vi "CoinDetector3.vi"() -> ()   [LabVIEW 2020]
uses:
  <vilib>/Analysis/5stat.llb/RMS (DBL).vi
  <vilib>/Analysis/NI_AALPro.lvlib
panel:
  in  "Boolean 3":bool
  in  "Boolean 2":bool
  in  "Boolean":bool
  out "7500 Hz":dbl
  out "6000 Hz":dbl
  out "3000 Hz":dbl
  out "data 2":dynamicdata(graph) caption="data"
  out "data":dynamicdata(graph)
  out "Freq":dbl
  out "Freq 2":dbl
  out "RMS2":dbl
  out "RMS":dbl
  in  "stop":bool
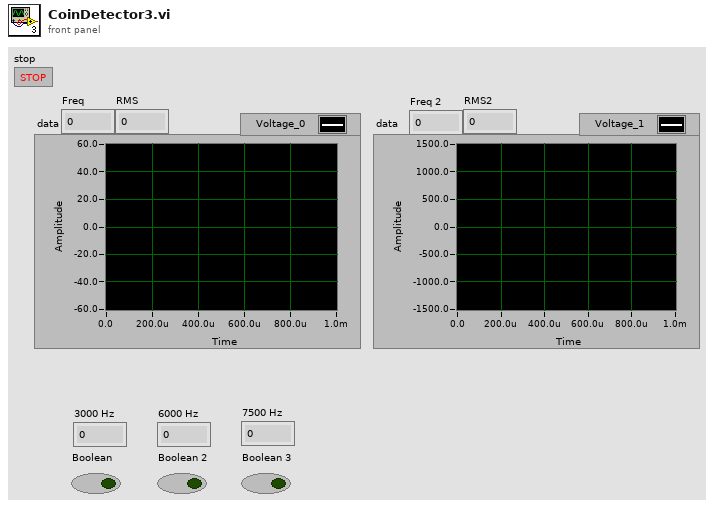
[diagram p1: front panel]
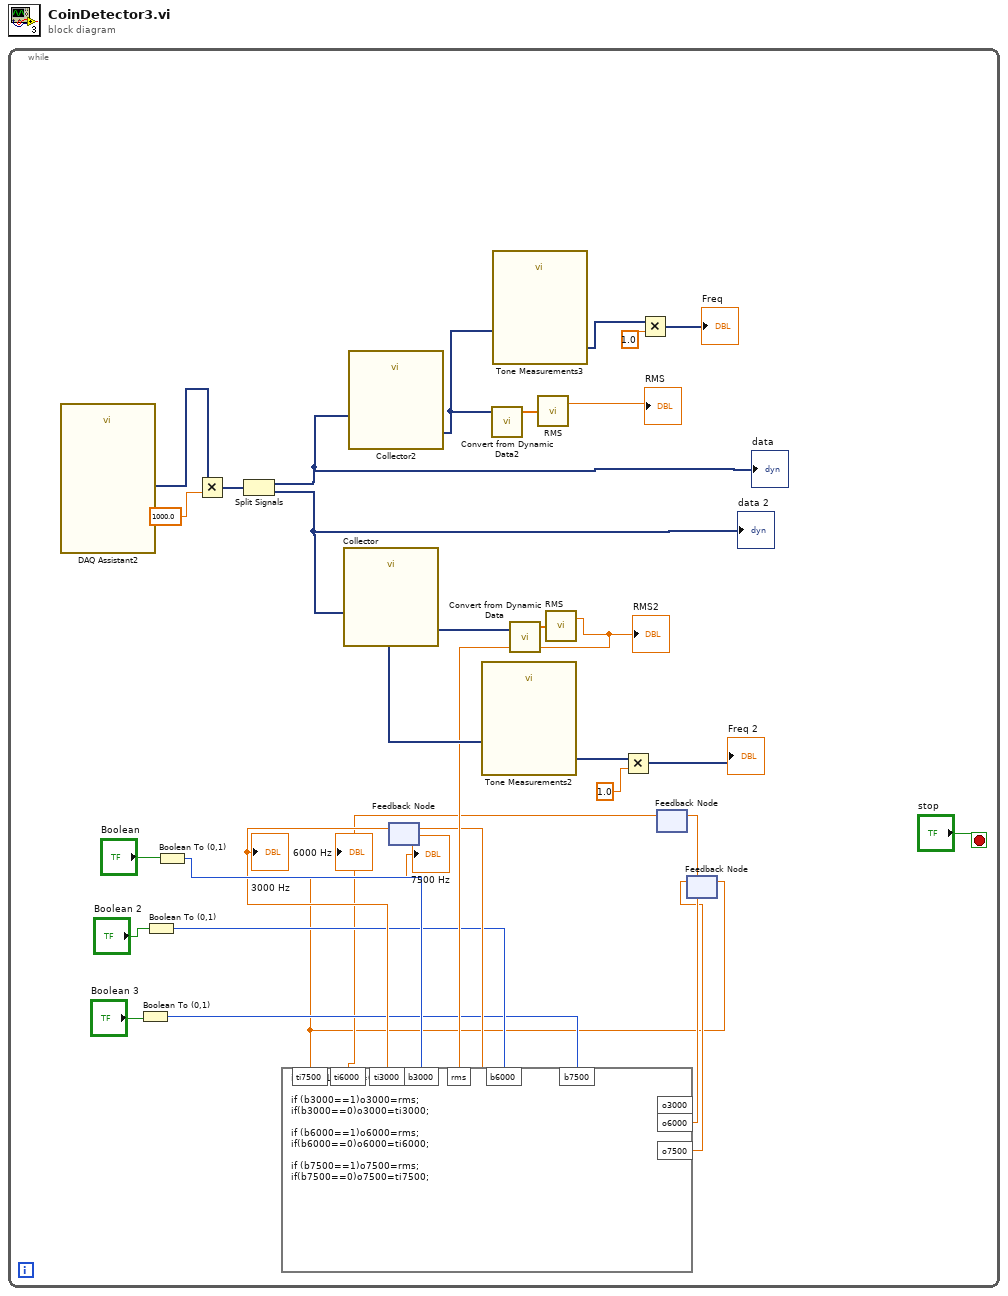
[diagram p0: block diagram]
diagram:
  n1 = while {
    stop <- "stop" stop-if-true
    n2 = call "DAQ Assistant2"() -> ("data"=w18:dynamicdata)  [unwired: 16 in, 3 out]
    n3 = Boolean To (0,1)(Boolean="Boolean 3") -> (0, 1=w5:i16)
    n4 = Boolean To (0,1)(Boolean="Boolean 2") -> (0, 1=w6:i16)
    n5 = Boolean To (0,1)(Boolean="Boolean") -> (0, 1=w12:i16)
    n6 = Multiply(x=w18, y=1000.0) -> (x*y=w28:dynamicdata)
    n7 = Split Signals(w28) -> (w15:dynamicdata, w14:dynamicdata)  [unwired: 2 in]
    "data" <- w15
    "data 2" <- w14
    n8 = call "Collector"("Signals"=w14) -> ("Collected Signals"=w17:dynamicdata)  [unwired: 9 in, 1 out]
    n9 = call "Collector2"("Signals"=w15) -> ("Collected Signals"=w22:dynamicdata)  [unwired: 9 in, 1 out]
    n10 = feedback #1() -> (w9:dbl)  [unwired: 1 in]
    "3000 Hz" <- w9
    n11 = call "Tone Measurements2"("Signals"=w17) -> ("Frequency"=w25:dynamicdata)  [unwired: 9 in, 1 out]
    n12 = call "Convert from Dynamic Data2"("Dynamic Data Type"=w22) -> ("Array"=w24:dbl[])  [unwired: 3 in]
    n13 = call "Tone Measurements3"("Signals"=w22) -> ("Frequency"=w21:dynamicdata)  [unwired: 9 in, 1 out]
    n14 = call "Convert from Dynamic Data"("Dynamic Data Type"=w17) -> ("Array"=w27:dbl[])  [unwired: 3 in]
    n15 = call-poly <vilib>:"RMS.vi"("X"=w24) -> ("rms value"=→"RMS":dbl)  [unwired: 1 out]
    n16 = call-poly <vilib>:"RMS.vi"("X"=w27) -> ("rms value"=w11:dbl)  [unwired: 1 out]
    "RMS2" <- w11
    n17 = Multiply(x=w25, y=1.0) -> (x*y=→"Freq 2":dynamicdata)
    n18 = Multiply(x=w21, y=1.0) -> (x*y=→"Freq":dynamicdata)
    n19 = feedback #2() -> (w3:dbl)  [unwired: 1 in]
    "6000 Hz" <- w3
    n20 = feedback #3() -> (w1:dbl)  [unwired: 1 in]
    "7500 Hz" <- w1
    n21 = formula code="int32 p1=0,p2=0,p3=0;\n\nif (b3000==1)o3000=rms;\nif(b3000==0)o3000=ti3000;\n\nif (b6000==1)o6000=rms;\nif(b6000==0)o6000=ti6000;\n\nif (b7500==1)o7500=rms;\nif(b7500==0)o7500=ti7500;"("b3000"=w12, "rms"=w11, "ti3000"=w9, "b6000"=w6, "b7500"=w5, "ti6000"=w3, "ti7500"=w1) -> ("o3000"=w10:dbl, "o6000"=w4:dbl, "o7500"=w2:dbl)
    n22 = feedback-in #1(w10) -> ()
    n23 = feedback-in #2(w4) -> ()
    n24 = feedback-in #3(w2) -> ()
  }
